vi "REQ Initialize Input.vi"(8 "error in (no error)":errorcluster, 9 "DAQ Type":enum16{"Hardware", "Simulation"}(ring), 10 "CAN Input":T1, 11 "PXI 8513 in":refnum<class "PXI 8513.lvclass">) -> (0 "error out":errorcluster, 3 "PXI 8513 out":refnum<class "PXI 8513.lvclass">)   [LabVIEW 2021, in "CAN.lvlib" / "PXI 8513.lvclass"]
uses:
  PXI 8513.lvclass
  CAN Input.ctl
  PXI 8513.lvclass/PXI 8513.ctl
  <vilib>/xnet/xnet.llb/XNET Create Session (Frame Input Stream).vi
  <resource>/objmgr/xnet.rc
  CAN.lvlib
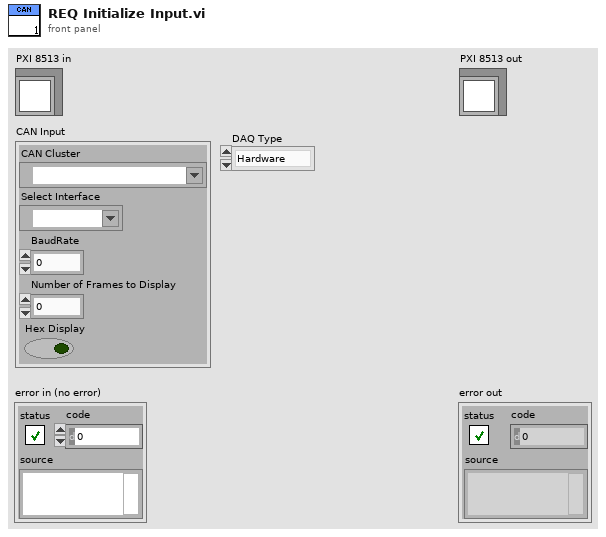
[diagram p1: front panel]
types:
  T1 = typedef "CAN.lvlib/CAN Input.ctl" = cluster{"CAN Cluster":refnum<k21>, "Select Interface":refnum<k21>, "BaudRate":u32, "Number of Frames to Display":i32, "Hex Display":bool}
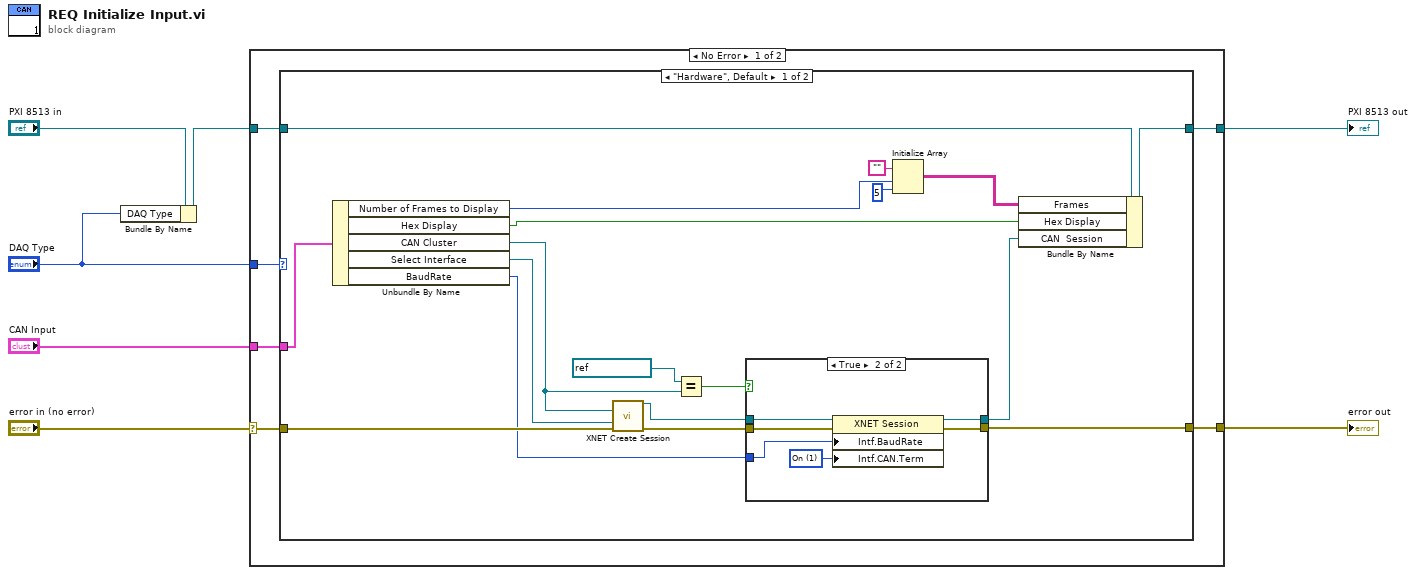
[diagram p0: block diagram]
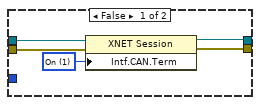
[diagram p2: hidden frame]
diagram:
  n1 = Bundle By Name(cluster="PXI 8513 in", "DAQ Type"="DAQ Type") -> (w4:refnum<class "PXI 8513.lvclass">)
  n2 = case shown="No Error" "error in (no error)" {
    selector: "error in (no error)" -> [w9 w45]
    tunnel: w4 -> [w12 w46]
    tunnel: [w11 w46] -> w5
    tunnel: "DAQ Type" -> [w13 _]
    tunnel: "CAN Input" -> [w10 _]
    tunnel: [w8 w45] -> w1
    frame No Error {
      n3 = case shown="\"Hardware\", Default" w13 {
        tunnel: w12 -> [w23 w44]
        tunnel: [w21 w44] -> w11
        tunnel: w10 -> [w28 _]
        tunnel: w9 -> [w30 w43]
        tunnel: [w19 w43] -> w8
        frame "Hardware", Default {
          n4 = Unbundle By Name(w28) -> ("Number of Frames to Display"=w14:i32, "Hex Display"=w15:bool, "CAN Cluster"=w26:refnum<k21>, "Select Interface"=w27:refnum<k21>, "BaudRate"=w24:u32)
          n5 = call-poly <vilib>:"XNET Create Session.vi"("cluster (:memory:)"=w26, "interface"=w27, "error in (no error)"=w30) -> ("session out"=w25:refnum<k21>, "error out"=w29:errorcluster)  [unwired: 11 out]
          n6 = Equal?(x=refnum<k21> ":memory:" ("CAN Cluster"), y=w26) -> (x = y?=w22:bool)
          n7 = case shown="True" w22 {
            tunnel: w29 -> [w35 w42]
            tunnel: w25 -> [w36 w41]
            tunnel: w24 -> [_ w40]
            tunnel: [w33 w38] -> w20
            tunnel: [w32 w37] -> w19
            frame False {
              w34 = u32 1 items=["Off", "On"] ("Interface:CAN:Termination")
              n8 = property class="XNET Session"(reference=w36, error in=w35, "Intf.CAN.Term"=w34) -> (reference out=w33:refnum<k21>, error out=w32:errorcluster)
            }
            frame True {
              w39 = u32 1 items=["Off", "On"] ("Interface:CAN:Termination")
              n9 = property class="XNET Session"(reference=w41, error in=w42, "Intf.BaudRate"=w40, "Intf.CAN.Term"=w39) -> (reference out=w38:refnum<k21>, error out=w37:errorcluster)
            }
          }
          n10 = Initialize Array("", w14, 5 ("Dimension Size")) -> (w16:string[][])
          n11 = Bundle By Name(cluster=w23, "Frames"=w16, "Hex Display"=w15, "CAN  Session"=w20) -> (w21:refnum<class "PXI 8513.lvclass">)
        }
        frame "Simulation" {
        }
      }
    }
    frame Error {
    }
  }
  "error out" <- w1
  "PXI 8513 out" <- w5
